vi "Pre Launch Init.vi"(11 "Main in":refnum<class "Main.lvclass">) -> (0 "error out":errorcluster, 3 "Main out":refnum<class "Main.lvclass">)   [LabVIEW 2024]
doc: "<p>(<strong>Filename</strong>: <span class=\"dnl\">Actor Framework.lvlib:Actor.lvclass:Pre Launch Init.vi</span>)</p>\n<p>Defines behavior that occurs after the <a href=\"nihelplauncher://docs/csh?context=lvcore_lvcomm_af_launch_nested_actor\">Launch Nested Actor</a> method is invoked but before the actor's Actor Core method begins running.</p>\n<p>By default, this method does nothing. A descendant class may override it to define behavior.</p>"
uses:
  Main.lvclass/Main.ctl
  Idle/Idle.lvclass
  State Actor/State Actor.lvclass
  C:/Users/ottoa/OneDrive/Desktop/working copies/stateActor/src/Sample State Actor/Main/Main.lvclass
  C:/Users/ottoa/OneDrive/Desktop/working copies/stateActor/src/State Actor/State Actor.lvclass
  C:/Program Files (x86)/National Instruments/LabVIEW 2024/vi.lib/ActorFramework/Actor/Actor.lvclass
  C:/Users/ottoa/OneDrive/Desktop/working copies/stateActor/src/Sample State Actor/Idle/Idle.lvclass
  Main.lvclass
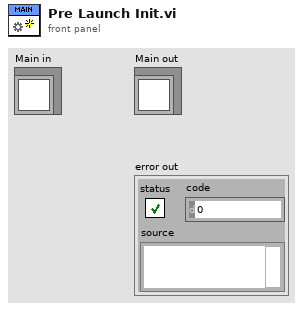
[diagram p1: front panel]
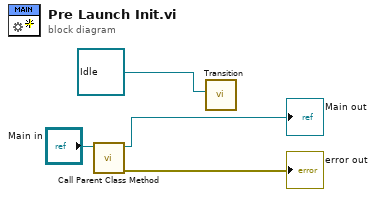
[diagram p0: block diagram]
diagram:
  n1 = call-parent "Call Parent Class Method"("State Actor in"="Main in") -> ("error out"=→"error out":errorcluster, "State Actor out"=→"Main out":refnum<class "Main.lvclass">)  [unwired: 9 in]
  n2 = call-dynamic "Transition.vi"("Target State Actor in"=refnum<class "Idle.lvclass"> refnum ("Sample State Actor.lvlib:Idle.lvclass")) -> ()  [unwired: 9 in, 2 out]
